vi "AverageSubarea_v1.vi"(9 "Pixel Width [um/pixel]":dbl, 10 "Selected Frame":dbl[][](graph), 11 "Positions":T1) -> (3 "mean":dbl format="%0.2f")   [LabVIEW 2010]
uses:
  <vilib>/Analysis/NI_AALBase.lvlib
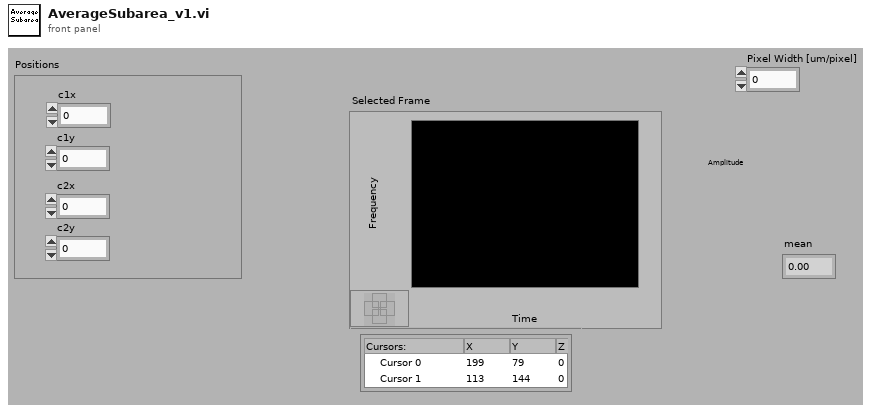
[diagram p1: front panel]
types:
  T1 = cluster{"c1x":dbl, "c1y":dbl, "c2x":dbl, "c2y":dbl}
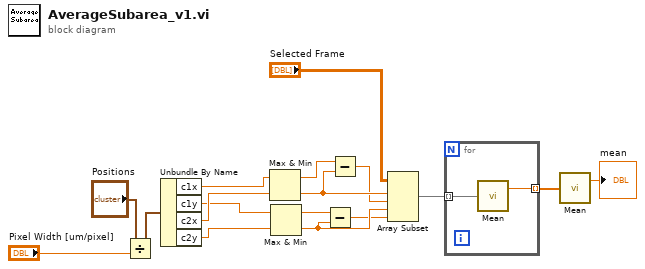
[diagram p0: block diagram]
diagram:
  n1 = Divide(x="Positions", y="Pixel Width [um/pixel]") -> (x/y=w1:T1)
  n2 = Unbundle By Name(w1) -> ("c1x"=w7:dbl, "c1y"=w5:dbl, "c2x"=w6:dbl, "c2y"=w4:dbl)
  n3 = Max & Min(x=w7, y=w6) -> (max(x,y)=w17:dbl, min(x,y)=w16:dbl)
  n4 = Max & Min(x=w5, y=w4) -> (max(x,y)=w14:dbl, min(x,y)=w13:dbl)
  n5 = Subtract(x=w14, y=w13) -> (x-y=w12:dbl)
  n6 = Subtract(x=w17, y=w16) -> (x-y=w15:dbl)
  n7 = Array Subset(array="Selected Frame", index (row)=w16, length (row)=w15, index (col)=w13, length (col)=w12) -> (w10:dbl[][])
  n8 = for {
    tunnel: w10 -> [w19] mode=indexing
    tunnel: [w18] -> w11 mode=indexing
    n9 = call <vilib>:"Mean.vi"("X"=w19) -> ("mean"=w18:dbl)  [unwired: 1 out]
  }
  n10 = call <vilib>:"Mean.vi"("X"=w11) -> ("mean"=→"mean":dbl)  [unwired: 1 out]
